vi "Write Waveforms.vi"(8 "error in (no error)":errorcluster, 10 "Waveforms":waveform(dbl)[](array[waveform]), 11 "FunctionBase in":refnum<class "FunctionBase.lvclass">) -> (0 "error out":errorcluster, 3 "FunctionBase out":refnum<class "FunctionBase.lvclass">)   [LabVIEW 2018, in "Functions.lvlib" / "FunctionBase.lvclass"]
uses:
  FunctionBase.lvclass
  FunctionBase.lvclass/FunctionBase.ctl
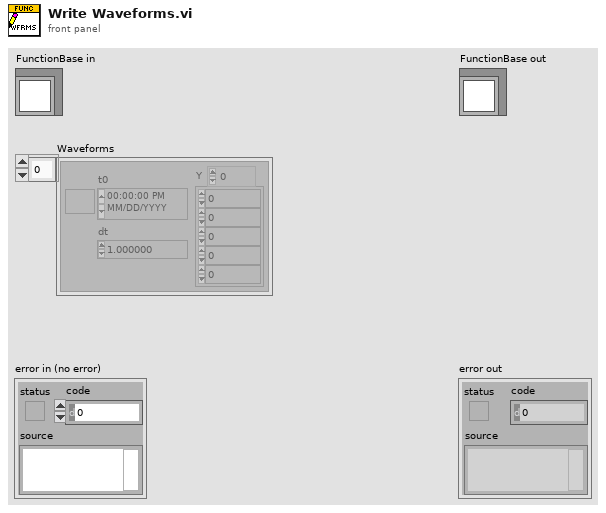
[diagram p1: front panel]
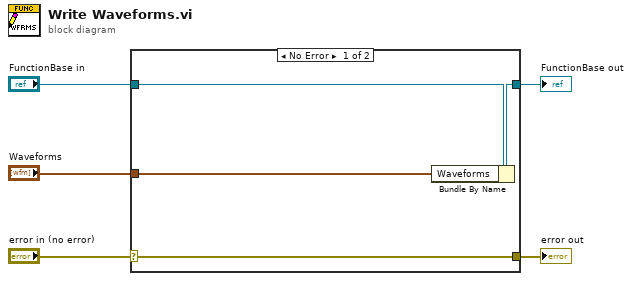
[diagram p0: block diagram]
diagram:
  n1 = case shown="No Error" "error in (no error)" {
    selector: "error in (no error)" -> [w9 w10]
    tunnel: [w9 w10] -> w4
    tunnel: [w7 w11] -> w2
    tunnel: "FunctionBase in" -> [w8 w11]
    tunnel: "Waveforms" -> [w6 _]
    frame No Error {
      n2 = Bundle By Name(cluster=w8, "Waveforms"=w6) -> (w7:refnum<class "FunctionBase.lvclass">)
    }
    frame Error {
    }
  }
  "error out" <- w4
  "FunctionBase out" <- w2
